vi "Log Measurment Configurations.vi"(0 "Data Cluster OUT in":T1 {"Measurement Configuration"."Relative To" items=["Power sequence start", "Previous source start", "Previous source end"]; "Measurement Configuration"."Power line frequency" items=["50 Hz", "60 Hz"]; "Measurement Configuration"."Start Value" format="%#_6p"; "Measurement Configuration"."Transient Response" items=["Slow", "Normal", "Fast"]; "Measurement Configuration"."Sense Mode" items=["Local Sense", "Remote Sense"]; "Measurement Configuration"."Target Value" format="%#_6p"; "Measurement Configuration"."Source Mode" items=["DC Voltage", "DC Current"]; "Measurement Configuration"."Start Delay" format="%#_6p"; "Measurement Configuration"."Compliance Limit" format="%#_6p"; "Measurement Configuration"."Ramp Rate" format="%#_6p"}, 1 "Cluster in":refnum<vi>, 3 "error in (no error)":errorcluster) -> (7 "Data Cluster OUT out":T1 {"Measurement Configuration"."Relative To" items=["Power sequence start", "Previous source start", "Previous source end"]; "Measurement Configuration"."Power line frequency" items=["50 Hz", "60 Hz"]; "Measurement Configuration"."Start Value" format="%#_6p"; "Measurement Configuration"."Transient Response" items=["Slow", "Normal", "Fast"]; "Measurement Configuration"."Sense Mode" items=["Local Sense", "Remote Sense"]; "Measurement Configuration"."Target Value" format="%#_6p"; "Measurement Configuration"."Source Mode" items=["DC Voltage", "DC Current"]; "Measurement Configuration"."Start Delay" format="%#_6p"; "Measurement Configuration"."Compliance Limit" format="%#_6p"; "Measurement Configuration"."Ramp Rate" format="%#_6p"}, 10 "error out":errorcluster)   [LabVIEW 2024, in "devicePowerSequencerCoreLogic.lvlib"]
doc: "Log Measurment Configurations"
uses:
  devicePowerSequencerCoreLogic.lvlib
  controls/Data Cluster.ctl
  <vilib>/Plug-In SDKs/Clients/Session Management V1/Session Reservation/Session Reservation.lvclass
  <vilib>/Plug-In SDKs/Measurements/Measure Call Context/Measure Call Context.lvclass
  Measurement Configuration.ctl
  controls/Source Mode.ctl
  controls/Sense Mode.ctl
  controls/Relative To.ctl
  controls/Transient Response.ctl
  controls/Power line frequency.ctl
  Measurement Results.ctl
  controls/Channel Name.ctl
  controls/Software Flags.ctl
  controls/Ramp Configurations.ctl
  controls/Error Info.ctl
  controls/Measurements.ctl
  controls/Voltage and Current Measurements.ctl
  controls/Log Configurations.ctl
  dataLogger/dataLogger.lvlib
  Device Power Sequencer.lvlib
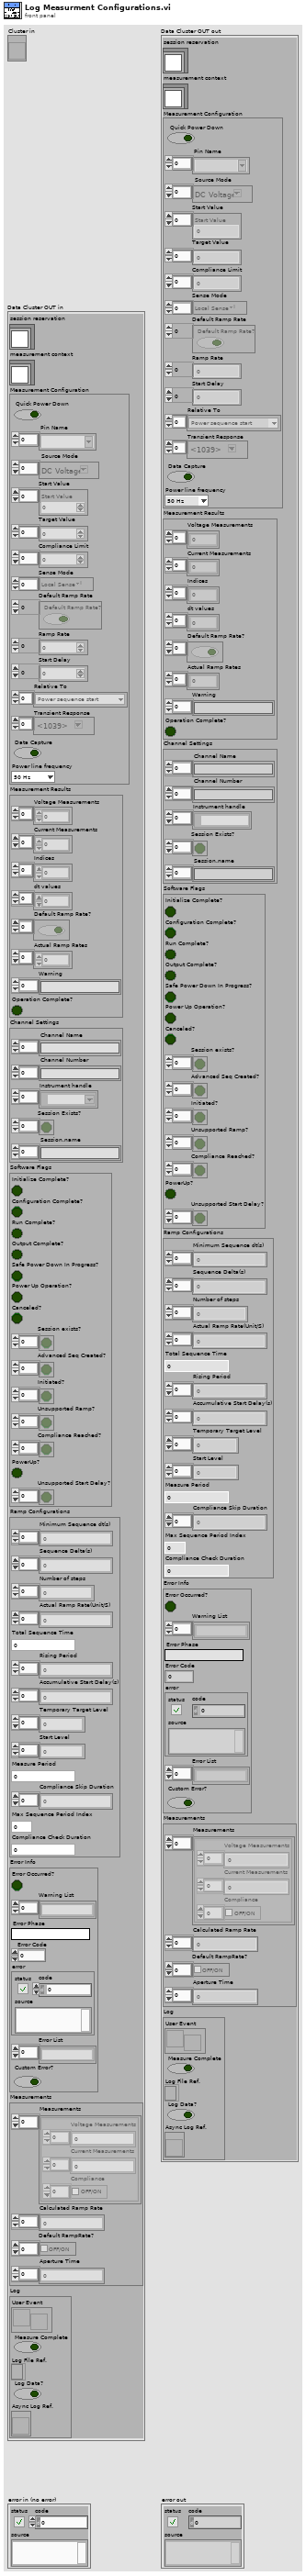
[diagram p1: front panel]
types:
  T1 = typedef "devicePowerSequencerCoreLogic.lvlib/Data Cluster.ctl" = cluster{"session reservation":refnum<class "Session Reservation.lvclass">, "measurement context":refnum<class "Measure Call Context.lvclass">, "Measurement Configuration":T2, "Measurement Results":T8, "Channel Settings":T9, "Software Flags":T10, "Ramp Configurations":T11, "Error Info":T12, "Measurements":T13, "Log":T15}
  T2 = typedef "Device Power Sequencer.lvlib/Measurement Configuration.ctl" = cluster{"Quick Power Down":bool, "Pin Name":string[], "Source Mode":T3[], "Start Value":dbl[], "Target Value":dbl[], "Compliance Limit":dbl[], "Sense Mode":T4[], "Default Ramp Rate":bool[], "Ramp Rate":dbl[], "Start Delay":dbl[], "Relative To":T5[], "Transient Response":T6[], "Data Capture":bool, "Power line frequency":T7}
  T3 = typedef "Device Power Sequencer.lvlib/Source Mode.ctl" = i32
  T4 = typedef "Device Power Sequencer.lvlib/Sense Mode.ctl" = i32
  T5 = typedef "Device Power Sequencer.lvlib/Relative To.ctl" = u32
  T6 = typedef "Device Power Sequencer.lvlib/Transient Response.ctl" = i32
  T7 = typedef "Device Power Sequencer.lvlib/Power line frequency.ctl" = u32
  T8 = typedef "Device Power Sequencer.lvlib/Measurement Results.ctl" = cluster{"Voltage Measurements":dbl[], "Current Measurements":dbl[], "Indices":i32[], "dt values":dbl[], "Default Ramp Rate?":bool[], "Actual Ramp Rates":dbl[], "Warning":string[], "Operation Complete?":bool}
  T9 = typedef "devicePowerSequencerCoreLogic.lvlib/Channel Name.ctl" = cluster{"Channel Name":string[], "Channel Number":string[], "Instrument handle":refnum<k15>[], "Session Exists?":bool[], "Session.name":string[]}
  T10 = typedef "devicePowerSequencerCoreLogic.lvlib/Software Flags.ctl" = cluster{"Initialize Complete?":bool, "Configuration Complete?":bool, "Run Complete?":bool, "Output Complete?":bool, "Safe Power Down In Progress?":bool, "Power Up Operation?":bool, "Canceled?":bool, "Session exists?":bool[], "Advanced Seq Created?":bool[], "Initiated?":bool[], "Unsupported Ramp?":bool[], "Compliance Reached?":bool[], "PowerUp?":bool, "Unsupported Start Delay?":bool[]}
  T11 = typedef "devicePowerSequencerCoreLogic.lvlib/Ramp Configurations.ctl" = cluster{"Minimum Sequence dt(s)":dbl[], "Sequence Delta(s)":dbl[], "Number of steps":i32[], "Actual Ramp Rate(Unit/S)":dbl[], "Total Sequence Time":dbl, "Rising Period":dbl[], "Accumulative Start Delay(s)":dbl[], "Temporary Target Level":dbl[], "Start Level":dbl[], "Measure Period":dbl, "Compliance Skip Duration":dbl[], "Max Sequence Period Index":i32, "Compliance Check Duration":dbl}
  T12 = typedef "devicePowerSequencerCoreLogic.lvlib/Error Info.ctl" = cluster{"Error Occurred?":bool, "Warning List":string[], "Error Phase":string, "Error Code":i32, "error":errorcluster, "Error List":string[], "Custom Error?":bool}
  T13 = typedef "devicePowerSequencerCoreLogic.lvlib/Measurements.ctl" = cluster{"Measurements":T14[], "Calculated Ramp Rate":dbl[], "Default RampRate?":bool[], "Aperture Time":dbl[]}
  T14 = typedef "devicePowerSequencerCoreLogic.lvlib/Voltage and Current Measurements.ctl" = cluster{"Voltage Measurements":dbl[], "Current Measurements":dbl[], "Compliance":bool[]}
  T15 = typedef "devicePowerSequencerCoreLogic.lvlib/Log Configurations.ctl" = cluster{"User Event":refnum<user-event>, "Measure Complete":bool, "Log File Ref.":refnum<file>, "Log Data?":bool, "Async Log Ref.":refnum<vi>}
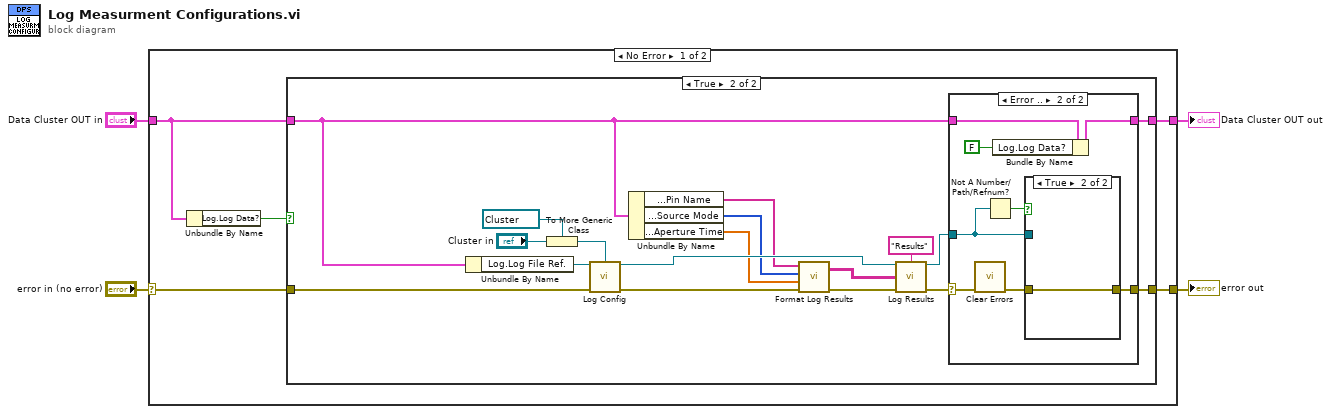
[diagram p0: block diagram]
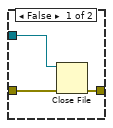
[diagram p4: hidden frame]
diagram:
  n1 = case shown="No Error" "error in (no error)" {
    selector: "error in (no error)" -> [w5 w44]
    tunnel: "Data Cluster OUT in" -> [w8 w45]
    tunnel: [w7 w45] -> w3
    tunnel: [w6 w44] -> w2
    frame No Error {
      n2 = Unbundle By Name(w8) -> ("Log.Log Data?"=w9:bool)
      n3 = case shown="True" w9 {
        tunnel: w5 -> [w10 w29]
        tunnel: w8 -> [w11 w15]
        tunnel: [w10 w14] -> w6
        tunnel: [w11 w16] -> w7
        frame False {
        }
        frame True {
          n4 = Unbundle By Name(w15) -> ("Log.Log File Ref."=w25:refnum<file>)
          n5 = To More Generic Class(target class=refnum<vi> refnum ("Measurement Configuration"), reference="Cluster in") -> (generic class reference=w26:refnum<vi>)
          n6 = call "Log Config.vi"("Log File Ref In"=w25, "Measurement Config Ref."=w26, "error in"=w29) -> ("Log File Ref Out"=w20:refnum<file>, "error out"=w23:errorcluster)  [unwired: 10 in, 1 out]
          n7 = Unbundle By Name(w15) -> ("Measurement Configuration.Pin Name"=w19:string[], "Measurement Configuration.Source Mode"=w18:T3[], "Measurements.Aperture Time"=w17:dbl[])
          n8 = call "Format Log Results.vi"("error in"=w23, "Aperture Time"=w17, "Source Mode"=w18, "Pin Name"=w19) -> ("error out"=w22:errorcluster, "Results"=w21:string[][])  [unwired: 6 in]
          n9 = call "Log Results.vi"("Log File Ref. In"=w20, "Results Name"="Results", "Data Input"=w21, "error in"=w22) -> ("Log File Ref. Out"=w12:refnum<file>, "error out"=w13:errorcluster)  [unwired: 9 in, 1 out]
          n10 = case shown="Error .." w13 {
            selector: w13 -> [w31 w38]
            tunnel: [w30 w37] -> w16
            tunnel: w15 -> [w30 w39]
            tunnel: [w31 w34] -> w14
            tunnel: w12 -> [_ w33]
            frame No Error {
            }
            frame Error {
              n11 = call <vilib>:"Clear Errors.vi"("error in (no error)"=w38) -> ("error out"=w35:errorcluster)  [unwired: 5 in, 1 out]
              n12 = Not A Number/Path/Refnum?(number/path/refnum=w33) -> (NaN/Path/Refnum?=w32:bool)
              n13 = Bundle By Name(cluster=w39, "Log.Log Data?"=FALSE) -> (w37:T1)
              n14 = case shown="True" w32 {
                tunnel: w35 -> [w42 w43]
                tunnel: [w41 w43] -> w34
                tunnel: w33 -> [w40 _]
                frame False {
                  n15 = Close File(refnum=w40, error in=w42) -> (error out=w41:errorcluster)  [unwired: 1 out]
                }
                frame True {
                }
              }
            }
          }
        }
      }
    }
    frame Error {
    }
  }
  "Data Cluster OUT out" <- w3
  "error out" <- w2
